vi "Update MB Sts Reg.vi"(8 "error in (no error)":errorcluster, 11 "Stand in":refnum<class "Stand.lvclass">) -> (0 "error out":errorcluster, 3 "Stand out":refnum<class "Stand.lvclass">)   [LabVIEW 2019, in "Stand.lvclass"]
uses:
  Stand.lvclass
  C:/Users/ANENKOV_V1/Desktop/src/Device_class/Device.lvclass
  Device_class/Device.lvclass/Device.ctl
  Stand.lvclass/Stand.ctl
  FPGA/TypeDef/DI index.ctl
  FPGA_API_class/FPGA API.lvclass/FPGA API.ctl
  FPGA_API_class/FPGA API.lvclass
  Device_class/Device.lvclass
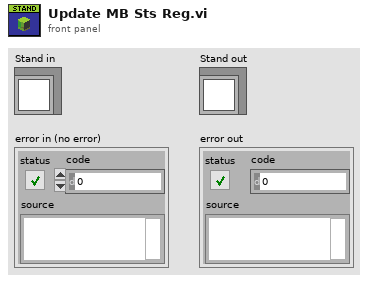
[diagram p1: front panel]
types:
  T1 = typedef "DI index.ctl" = u8
  T2 = typedef "STS REG.ctl" = cluster{"IDLE":bool, "RYADY":bool, "STEP":bool, "ALARM":bool, "WARNING":bool, "REMOTE":bool, "SP_EXEC_DONE_DUT":bool, "SP_EXEC_DONE_CHAMBER":bool, "FILING_DONE_DUT":bool, "FILING_DONE_CHAMBER":bool, "BURETE_STATE":bool}
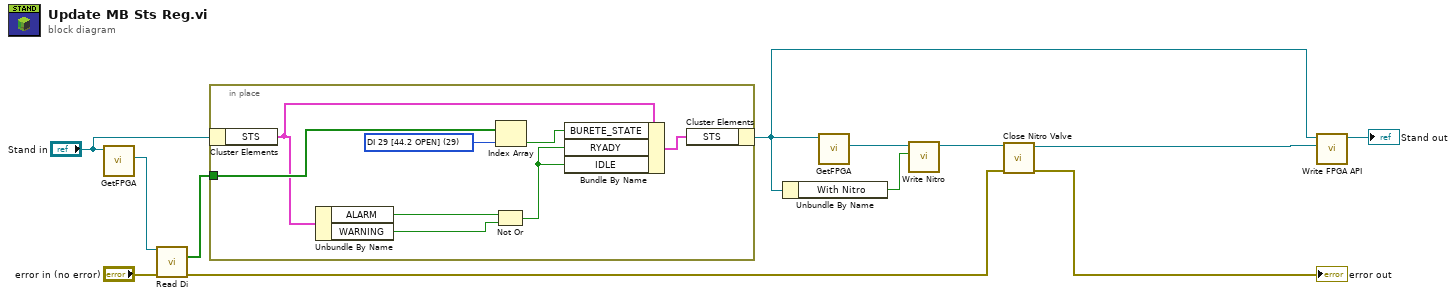
[diagram p0: block diagram]
diagram:
  n1 = call "GetFPGA.vi"("Device in"="Stand in") -> ("FPGA API.lvclass"=w11:refnum<class "FPGA API.lvclass">)  [unwired: 10 in]
  n2 = call-dynamic "Read Di.vi"("FPGA API in"=w11, "error in (no error)"="error in (no error)") -> ("DIs"=w9:bool[], "error out"=w2:errorcluster)  [unwired: 11 in, 1 out]
  n3 = in-place {
    in-place-border: w9 -> [w19]
    w18 = T1 29 items=["DI 0 [QF1]", "DI 1 [QF2]", "DI 2 [QF3]", "DI 3 [QF4]", "DI 4 [QF5]", "DI 5 [QF6]", "DI 6 [QF7]", "DI 7 [QF8]", "DI 8 [QF9]", "DI 9 [PHASE CONTROL RELAY CONTACTOR [KV1]]", "DI 10 [G1]", "DI 11 [G2]", "DI 12 [RESET BTN [SB1]]", "DI 13 [START BTN [SB2]]", "DI 14 [STOP BTN [SB3]]", "DI 15 [ES BTN [SB4]]", "DI 16 [MANUAL/AUTO MODE SA1]", "DI 17 [[S1]]", "DI 18 [[S2]]", "DI 19 [[S3]]", "DI 20 [[S4]]", "DI 21 [44.1 OPEN]", "DI 22 [44.1 CLOSE]", "DI 23 [CONTACTOR [MK1]] M12", "DI 24 [AUTOMATIC [QF11]] M12", "DI 25 [CONTACTOR [MK2]] M21", "DI 26 [AUTOMATIC [QF12]] M21", "DI 27 [CONTACTOR [MK3]] M24", "DI 28 [AUTOMATIC [QF13]] M24", "DI 29 [44.2 OPEN]", "DI 30 [44.2 CLOSE]"] ("DI index")
    n4 = in-place-cluster #1("Stand in") -> ("STS"=w16:T2)
    n5 = Unbundle By Name(w16) -> ("ALARM"=w15:bool, "WARNING"=w14:bool)
    n6 = Not Or(1:w14, 2:w15) -> (0:w13:bool)
    n7 = Index Array(array=w19, index=w18) -> (element=w17:bool)
    n8 = Bundle By Name(cluster=w16, "BURETE_STATE"=w17, "RYADY"=w13, "IDLE"=w13) -> (w20:T2)
    n9 = in-place-cluster #1("STS"=w20) -> (w6:refnum<class "Stand.lvclass">)
  }
  n10 = Unbundle By Name(w6) -> ("With Nitro"=w3:bool)
  n11 = call "GetFPGA.vi"("Device in"=w6) -> ("FPGA API.lvclass"=w7:refnum<class "FPGA API.lvclass">)  [unwired: 10 in]
  n12 = call "Write Nitro.vi"("Nitro"=w3, "FPGA API in"=w7) -> ("FPGA API out"=w5:refnum<class "FPGA API.lvclass">)  [unwired: 9 in]
  n13 = call-dynamic "Close Nitro Valve.vi"("error in (no error)"=w2, "FPGA API in"=w5) -> ("error out"=→"error out":errorcluster, "FPGA API out"=w4:refnum<class "FPGA API.lvclass">)  [unwired: 8 in]
  n14 = call "Write FPGA API.vi"("FPGA API.lvclass"=w4, "Device in"=w6) -> ("Device out"=→"Stand out":refnum<class "Stand.lvclass">)  [unwired: 9 in]
